vi "ImgRealAddTool.vi"(10 "ToolData":cluster{"X":dbl, "Y":dbl, "Angle":dbl}={"X"=-45.8415, "Y"=-15.9295, "Angle"=0.0}, 11 "ImgRealData":T1={"x imgreal"=-45.8415, "y imgreal"=-15.9295, "VisionAngle"=0.0}) -> (2 "YFinal":dbl, 3 "XFinal":dbl)   [LabVIEW 2019]
uses:
  <vilib>/Analysis/coordinate.llb/2D Cartesian Coordinate Rotation (Scalar).vi
  <vilib>/Analysis/NI_AALPro.lvlib
panel:
  out "y out":dbl
  out "x out":dbl
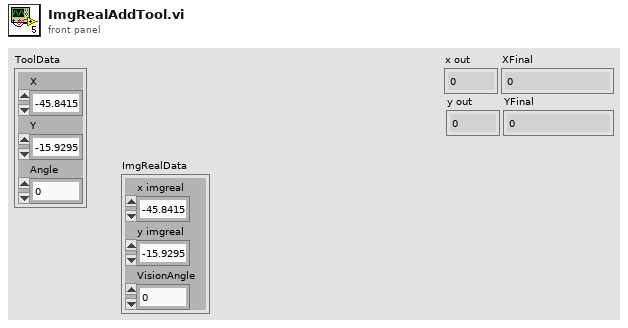
[diagram p1: front panel]
types:
  T1 = cluster{"x imgreal":dbl, "y imgreal":dbl, "VisionAngle":dbl}
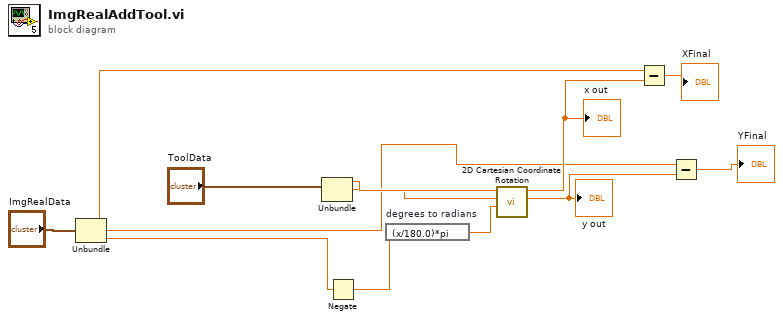
[diagram p0: block diagram]
diagram:
  n1 = Unbundle("ImgRealData") -> ("x imgreal"=w1:dbl, "y imgreal"=w2:dbl, "VisionAngle"=w3:dbl)
  n2 = Unbundle("ToolData") -> ("X"=w12:dbl, "Y"=w11:dbl)  [unwired: 1 out]
  n3 = Negate(x=w3) -> (-x=w5:dbl)
  n4 = expression code="(x/180.0)*pi" "degrees to radians"(w5) -> (w10:dbl)
  n5 = call-poly <vilib>:"2D Cartesian Coordinate Rotation.vi"("theta"=w10, "y"=w11, "x"=w12) -> ("y out"=w7:dbl, "x out"=w9:dbl)  [unwired: 6 in, 1 out]
  "x out" <- w9
  "y out" <- w7
  n6 = Subtract(x=w1, y=w9) -> (x-y=→"XFinal":dbl)
  n7 = Subtract(x=w2, y=w7) -> (x-y=→"YFinal":dbl)
